vi "User Access Level FGV.vi"(7 "User Access Level Cmd":T1, 8 "Error In":errorcluster, 10 "User Name":string) -> (0 "Error Out":errorcluster, 1 "User Level":string)   [LabVIEW 2017]
doc: "This FGV holds the Access Level for the user currently logged in. It executes the following methods:\n\n1. <B>Read User Access Level File:</B> Reads a tab-delimited text file containing User Names and corresponding Access Levels.\n2. <B>Set Current Access Level:</B> Sets the Access level for the User Name input.\n3. <B>Get Current Access Level:</B> Returns the Access level for the current User."
uses:
  User Level Cmd.ctl
  <vilib>/Utility/file.llb/Read Delimited Spreadsheet (string).vi
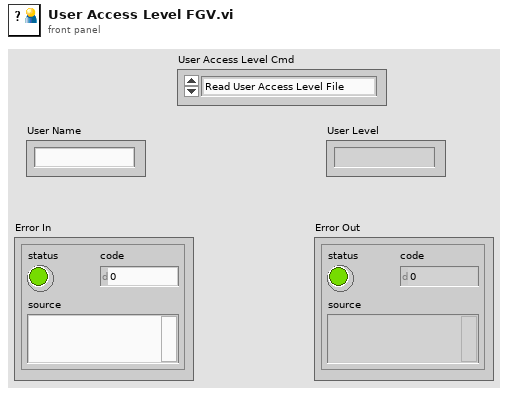
[diagram p1: front panel]
types:
  T1 = typedef "User Level Cmd.ctl" = enum16{"Read User Access Level File", "Set Current User", "Get User Access Level"}
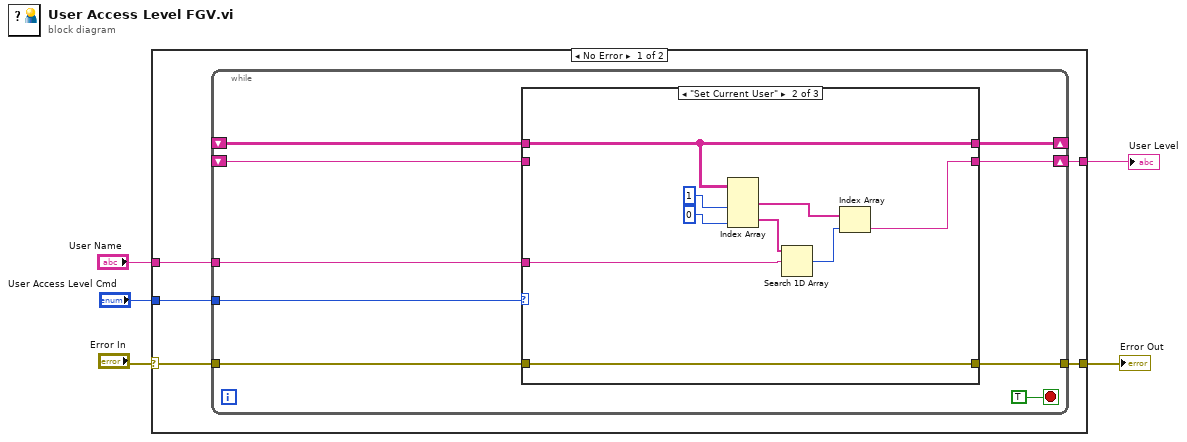
[diagram p0: block diagram]
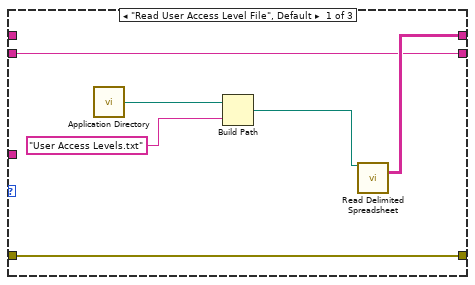
[diagram p2: hidden frame]
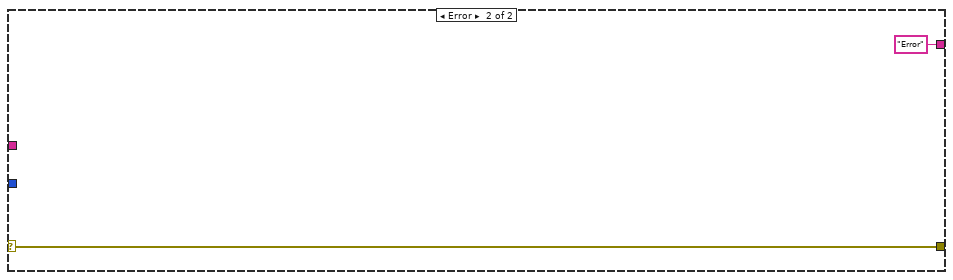
[diagram p4: hidden frame]
diagram:
  n1 = case shown="No Error" "Error In" {
    selector: "Error In" -> [w8 w39]
    tunnel: "User Access Level Cmd" -> [w10 _]
    tunnel: [w9 w39] -> w3
    tunnel: "User Name" -> [w7 _]
    tunnel: [w6 "Error" ("String")] -> w1
    frame No Error {
      n2 = while {
        tunnel: w10 -> [w19]
        tunnel: [w18] -> w9
        tunnel: w8 -> [w17]
        shift-right: [w15] -> _
        shift-left: _ -> [w14]
        tunnel: w7 -> [w13]
        shift-right: [w12] -> w6
        shift-left: _ -> [w11]
        stop <- TRUE stop-if-true
        n3 = case shown="\"Set Current User\"" w19 {
          tunnel: [w20 w34 w35] -> w18
          tunnel: w17 -> [w20 w34 w35]
          tunnel: [w22 w33 w37] -> w15
          tunnel: w14 -> [_ w33 w37]
          tunnel: w13 -> [_ w26 _]
          tunnel: [w21 w29 w36] -> w12
          tunnel: w11 -> [w21 _ w36]
          frame "Read User Access Level File", Default {
            n4 = call <vilib>:"Application Directory.vi"() -> ("Application Directory"=w24:path)
            n5 = Build Path(base path=w24, name or relative path="User Access Levels.txt") -> (appended path=w23:path)
            n6 = call-poly <vilib>:"Read Delimited Spreadsheet.vi"("file path (dialog if empty)"=w23) -> ("all rows"=w22:string[][])  [unwired: 9 in, 5 out]
          }
          frame "Set Current User" {
            n7 = Index Array(array=w33, index (col) #1=1 ("index (row)"), index (col) #2=0 ("index (row)")) -> (element #1=w31:string[], element #2=w32:string[])  [unwired: 2 in]
            n8 = Search 1D Array(1D array=w32, element=w26) -> (index of element=w30:i32)  [unwired: 1 in]
            n9 = Index Array(array=w31, index=w30) -> (element=w29:string)
          }
          frame "Get User Access Level" {
          }
        }
      }
    }
    frame Error {
    }
  }
  "User Level" <- w1
  "Error Out" <- w3
